vi "Add Subaddress.vi"(7 "error in":errorcluster, 8 "direction":T1, 9 "subaddress":T2, 10 "remote terminal":T3 format="%.0x") -> (0 "error out":errorcluster, 2 "subaddress section":T3 format="%.0x", 3 "remote terminal out":T3 format="%.0x")   [LabVIEW 2023, in "Ballard MIL-STD-1553 Scripting.lvlib"]
uses:
  Ballard MIL-STD-1553 Scripting.lvlib
  <vilib>/NI VeriStand/Custom Device API/Custom Device Item Ref.ctl
  Shared/Address.ctl
  Shared/Direction.ctl
  Constants.vi
  <vilib>/NI VeriStand/Custom Device API/Custom Device API.lvlib
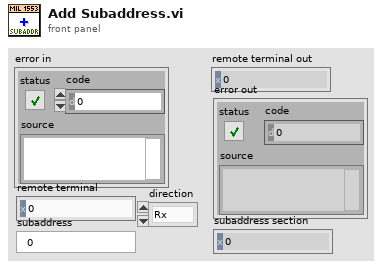
[diagram p1: front panel]
types:
  T1 = typedef "Direction.ctl" = enum16{"Rx", "Tx"}
  T2 = typedef "Address.ctl" = u16
  T3 = typedef "Custom Device API.lvlib/Custom Device Item Ref.ctl" = u64
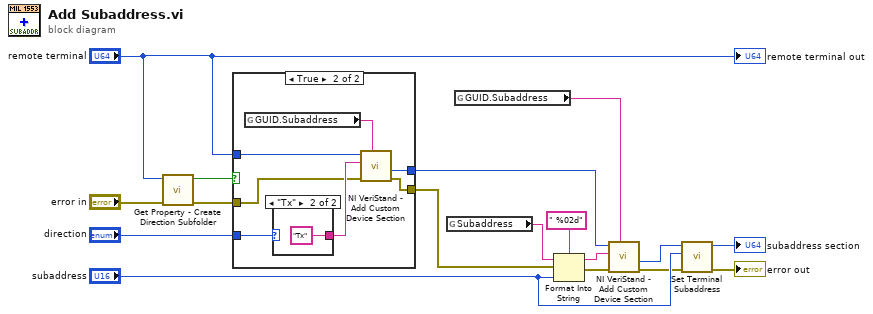
[diagram p0: block diagram]
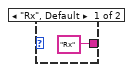
[diagram p3: hidden frame]
diagram:
  n1 = call "Get Property - Create Direction Subfolder.vi"("error in"="error in", "custom device"="remote terminal") -> ("error out"=w10:errorcluster, "Value"=w9:bool)  [unwired: 8 in]
  n2 = case shown="True" w9 {
    tunnel: "direction" -> [_ w26]
    tunnel: w10 -> [w19 w24]
    tunnel: [w19 w23] -> w13
    tunnel: "remote terminal" -> [w18 w22]
    tunnel: [w18 w21] -> w12
    frame False {
    }
    frame True {
      n3 = global read "Constants.vi" "GUID.Subaddress"() -> (w20:string)
      n4 = case shown="\"Tx\"" w26 {
        tunnel: ["Rx" "Tx"] -> w25
        frame "Rx", Default {
        }
        frame "Tx" {
        }
      }
      n5 = call <vilib>:"NI VeriStand - Add Custom Device Section.vi"("GUID (Default Section)"=w20, "error in (no error)"=w24, "Section Name"=w25, "Parent Ref in"=w22) -> ("error out"=w23:errorcluster, "Section Ptr"=w21:T3)  [unwired: 4 in, 2 out]
    }
  }
  n6 = global read "Constants.vi" "Subaddress"() -> (w6:string)
  n7 = global read "Constants.vi" "GUID.Subaddress"() -> (w7:string)
  n8 = Format Into String(format string=" %02d", initial string=w6, error in=w13, "subaddress") -> (resulting string=w16:string, error out=w15:errorcluster)
  n9 = call <vilib>:"NI VeriStand - Add Custom Device Section.vi"("GUID (Default Section)"=w7, "error in (no error)"=w15, "Section Name"=w16, "Parent Ref in"=w12) -> ("error out"=w3:errorcluster, "Section Ptr"=w5:T3)  [unwired: 4 in, 2 out]
  n10 = call "Set Terminal Subaddress.vi"("error in"=w3, "subaddress"="subaddress", "subaddress in"=w5) -> ("error out"=→"error out":errorcluster, "subaddress out"=→"subaddress section":T3)  [unwired: 7 in]
  "remote terminal out" <- "remote terminal"
